vi "Audio Analyzer Demo.vi"() -> ()   [LabVIEW 2019]
uses:
  <vilib>/Memosfet/myRIO-Neopixel/RT/Display Utilities/Public/Controls/2D Dimensions.ctl
  <vilib>/Memosfet/myRIO-Neopixel/RT/Graph/Graph.lvclass
  C:/Program Files (x86)/National Instruments/LabVIEW 2019/vi.lib/Memosfet/myRIO-Neopixel/RT/Display Element/Display Element.lvclass
  <vilib>/Memosfet/myRIO-Neopixel/RT/Graph/Public/Controls/Fill To.ctl
  <vilib>/Memosfet/myRIO-Neopixel/RT/Graph/Public/Controls/Range.ctl
  <vilib>/Memosfet/myRIO-Neopixel/RT/Display/Public/Controls/RGB Gains.ctl
  <vilib>/FPGAPlugInAG/myRIO-1900/niLvFpga_Open_myRIO-1900.vi
  <vilib>/rvi/interface/common/dynamic/niFpgaDynamicAddResources.vi
  <vilib>/FPGAPlugInAG/Dynamic/niLvFpga_Reset_Dynamic.vi
  <vilib>/Utility/error.llb/Error Cluster From Error Code.vi
  <vilib>/rvi/errors/niLvFpgaAdjustHostInterfaceError.vi
  <vilib>/rvi/Analysis/host/Private/Sample Rate To Loop Time (ticks).vi
  <vilib>/FPGAPlugInAG/Dynamic/niLvFpga_Close_Dynamic.vi
  <vilib>/rvi/interface/nirviOpenFPGA/nirviOpenFPGA.xnode
  Bitfiles/mydashboard_FPGATarget_MainFPGA1_sclqAr1bu20.lvbitx
  <vilib>/rvi/interface/nirviMethod/nirviMethod.xnode
  <vilib>/rvi/interface/nirviReadWriteControl/nirviReadWriteControl.xnode
  <vilib>/rvi/interface/nirviCloseFPGA/nirviCloseFPGA.xnode
  <vilib>/Memosfet/myRIO-Neopixel/RT/Display/Display.lvclass
  <vilib>/rvi/Analysis/host/Public/NI_FpgaMspHost.lvlib
  <vilib>/FPGAPlugInAG/Dynamic/niLvFpga_ReadFifo_Dynamic.vi
  <vilib>/rvi/errors/niLvFpgaMergeErrorWithErrorCode.vi
  <vilib>/Memosfet/myRIO-Neopixel/RT/Display Utilities/Display Utilities.lvlib
  NiFpgaLv.dll
  <vilib>/rvi/interface/Simulation/niFpgaSimulationCallBeginRW.vi
  <vilib>/FPGAPlugInAG/Dynamic/niLvFpga_WriteFifo_Dynamic.vi
panel:
  out "Error Out":errorcluster
  in  "Gain":sgl(slide)=0.45627376 scale=0.0..1.0
  in  "Stop":bool
  out "Invalid Sample Rate":bool
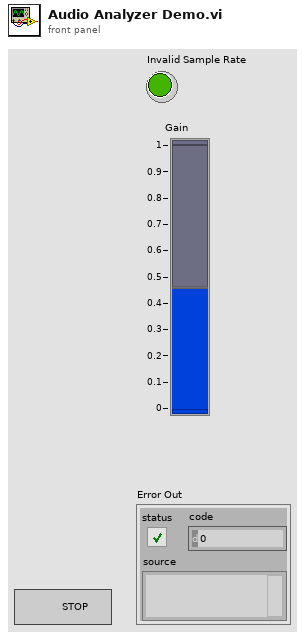
[diagram p1: front panel]
types:
  T1 = typedef "Graph.lvclass/Range.ctl" = cluster{"Maximum":dbl, "Minimum":dbl}
  T2 = typedef "Graph.lvclass/Fill To.ctl" = enum16{"None", "Inf", "-Inf"}
  T3 = typedef "Display Utilities.lvlib/2D Dimensions.ctl" = cluster{"Width":i32, "Height":i32}
  T4 = typedef "Display.lvclass/RGB Gains.ctl" = cluster{"Red":sgl, "Green":sgl, "Blue":sgl}
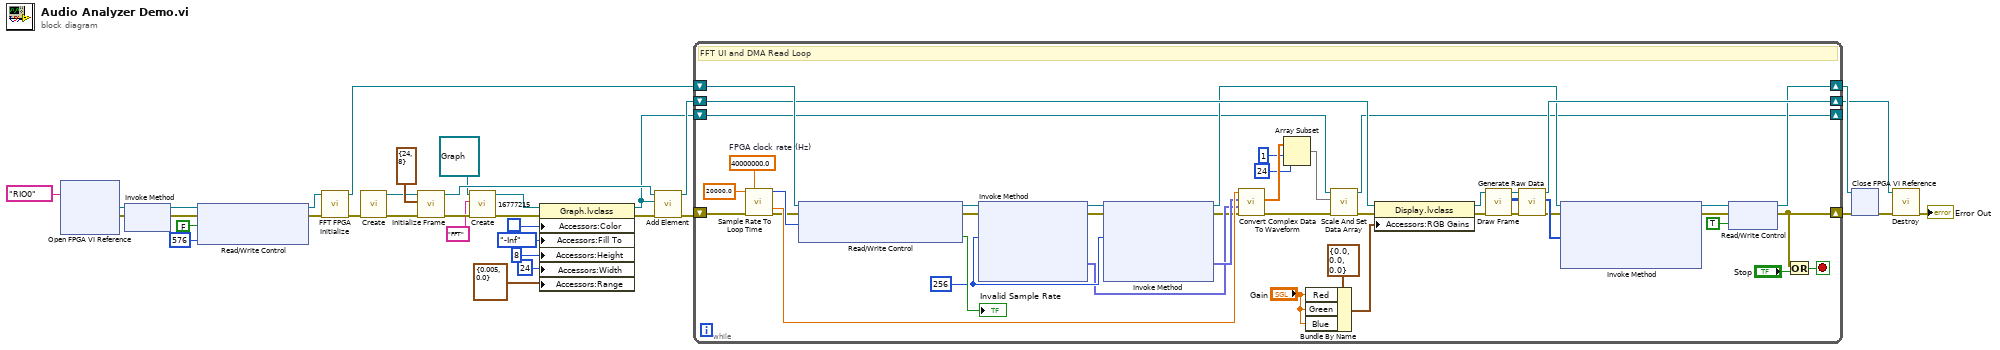
[diagram p0: block diagram]
diagram:
  n1 = xnode "Open FPGA VI Reference"("resource name"=tag "RIO0") -> ("FPGA VI Reference Out"=w30:refnum<k20>, "error out"=w31:errorcluster)  [unwired: 1 in]
  n2 = xnode "Invoke Method"("FPGA VI Reference In"=w30, "error in"=w31) -> ("FPGA VI Reference Out"=w7:refnum<k20>, "error out"=w6:errorcluster)
  n3 = xnode "Read/Write Control"("FPGA VI Reference In"=w7, "error in"=w6, "Update"=FALSE, "Number Of Elements"=576) -> ("FPGA VI Reference Out"=w3:refnum<k20>, "error out"=w4:errorcluster)
  n4 = call "FFT FPGA Initialize.vi"("error in (no error)"=w4, "Refnum in"=w3) -> ("error out"=w21:errorcluster, "Refnum out"=w32:refnum<k20>)  [unwired: 8 in]
  n5 = call <vilib>:"Create.vi"("Error In"=w21) -> ("Error Out"=w26:errorcluster, "Screen Out"=w27:refnum<class "Display.lvclass">)  [unwired: 9 in]
  n6 = call <vilib>:"Initialize Frame.vi"("Error In"=w26, "Size"=T3 {"Width"=24, "Height"=8}, "Display In"=w27) -> ("Error Out"=w25:errorcluster, "Display Out"=w24:refnum<class "Display.lvclass">)  [unwired: 7 in]
  n7 = call-dynamic <vilib>:"Create.vi"("Error In"=w25, "Tag"="FFT", "Graph In"=refnum<class "Graph.lvclass"> refnum) -> ("Error Out"=w15:errorcluster, "Graph Out"=w16:refnum<class "Graph.lvclass">)  [unwired: 7 in]
  n8 = property class="Graph.lvclass"(reference=w16, error in=w15, "Accessors:Color"=u32 16777215 ("Color"), "Accessors:Fill To"=Fill_To."-Inf" ("Fill To"), "Accessors:Height"=u32 8 ("Height"), "Accessors:Width"=u32 24 ("Width"), "Accessors:Range"=T1 {"Maximum"=0.005, "Minimum"=0.0} ("Range")) -> (reference out=w9:refnum<class "Graph.lvclass">, error out=w14:errorcluster)
  n9 = call <vilib>:"Add Element.vi"("Error In"=w14, "New Element"=w9, "Display In"=w24) -> ("Error Out"=w20:errorcluster, "Display Out"=w19:refnum<class "Display.lvclass">)  [unwired: 7 in]
  n10 = while {
    shift-right: [w46] -> w34
    shift-left: w32 -> [w68]
    shift-right: [w45] -> w33
    shift-left: w20 -> [w69]
    shift-right: [w60] -> w18
    shift-left: w19 -> [w58]
    shift-right: [w40] -> _
    shift-left: w9 -> [w42]
    stop <- w76 stop-if-true
    w72 = u32 256 ("Number of Elements")
    w67 = 40000000.0  # FPGA clock rate (Hz)
    # "FFT UI and DMA Read Loop"
    n11 = call-poly <vilib>:"Sample Rate To Loop Time.vi"("sample rate (S/s)"=20000.0 ("Sample rate (S/s)"), "FPGA clock rate (Hz)"=w67, "error in (no error)"=w69) -> ("count (ticks/S)"=w66:u32, "actual sample rate (S/s)"=w65:dbl, "error out"=w61:errorcluster)  [unwired: 10 in]
    n12 = xnode "Read/Write Control"("FPGA VI Reference In"=w68, "error in"=w61, "Requested Sample Period (ticks)"=w66) -> ("FPGA VI Reference Out"=w75:refnum<k20>, "error out"=w70:errorcluster, "Invalid Period"=→"Invalid Sample Rate":bool)
    n13 = xnode "Invoke Method"("FPGA VI Reference In"=w75, "error in"=w70, "Number of Elements"=w72) -> ("FPGA VI Reference Out"=w78:refnum<k20>, "error out"=w71:errorcluster, "Data"=w63:fxp<+/-,25,14>[])  [unwired: 1 in, 1 out]
    n14 = xnode "Invoke Method"("FPGA VI Reference In"=w78, "error in"=w71, "Number of Elements"=w72) -> ("FPGA VI Reference Out"=w50:refnum<k20>, "error out"=w62:errorcluster, "Data"=w64:fxp<+/-,25,14>[])  [unwired: 1 in, 1 out]
    n15 = call "Convert Complex Data To Waveform.vi"("error in"=w62, "Real Data"=w63, "Imaginary Data"=w64, "Sample Rate (S/s)"=w65) -> ("error out"=w41:errorcluster, "spectrum out"=w38:dbl[])  [unwired: 5 in, 1 out]
    n16 = Array Subset(array=w38, index=1, length=24) -> (w37:dbl[])
    n17 = Bundle By Name(cluster=T4 {"Red"=0.0, "Green"=0.0, "Blue"=0.0} ("RGB Gains"), "Red"="Gain", "Green"="Gain", "Blue"="Gain") -> (w53:T4)
    n18 = call <vilib>:"Scale And Set Data Array.vi"("Error In"=w41, "Data Array"=w37, "Graph In"=w42) -> ("Error Out"=w39:errorcluster, "Graph Out"=w40:refnum<class "Graph.lvclass">)  [unwired: 7 in]
    n19 = property class="Display.lvclass"(reference=w58, error in=w39, "Accessors:RGB Gains"=w53) -> (reference out=w57:refnum<class "Display.lvclass">, error out=w56:errorcluster)
    n20 = call <vilib>:"Draw Frame.vi"("Error In"=w56, "Display In"=w57) -> ("Error Out"=w51:errorcluster, "Frame"=w43:u32[][], "Display Out"=w52:refnum<class "Display.lvclass">)  [unwired: 7 in]
    n21 = call <vilib>:"Generate Raw Data.vi"("Error In"=w51, "Matrix"=w43, "Display In"=w52) -> ("Error Out"=w49:errorcluster, "Raw Data"=w59:u8[], "Display Out"=w60:refnum<class "Display.lvclass">)  [unwired: 6 in]
    n22 = xnode "Invoke Method"("FPGA VI Reference In"=w50, "error in"=w49, "Data"=w59) -> ("FPGA VI Reference Out"=w47:refnum<k20>, "error out"=w48:errorcluster)  [unwired: 1 in, 1 out]
    n23 = xnode "Read/Write Control"("FPGA VI Reference In"=w47, "error in"=w48, "Update"=TRUE) -> ("FPGA VI Reference Out"=w46:refnum<k20>, "error out"=w45:errorcluster)
    n24 = Or(x=w45, y="Stop") -> (x .or. y?=w76:bool)
  }
  n25 = xnode "Close FPGA VI Reference"("FPGA VI Reference In"=w34, "error in"=w33) -> ("error out"=w17:errorcluster)
  n26 = call <vilib>:"Destroy.vi"("Error In"=w17, "Display In"=w18) -> ("Error Out"=→"Error Out":errorcluster)  [unwired: 9 in]
